vi "Actor Core.vi"(8 "error in":errorcluster, 11 "Power Meter Display in":refnum<class "Power Meter Display.lvclass">) -> (0 "error out":errorcluster, 3 "Actor out":refnum<class "Actor.lvclass">)   [LabVIEW 2013, in "Display Panel.lvlib" / "Power Meter Display.lvclass"]
doc: "(<B>Filename</B>: Actor Framework.lvlib:Actor.lvclass:Actor Core.vi)\n\nReceives messages to the actor, reacts to them, and initiates any error handling that may shut the actor down.\n\nDescendant classes may override this VI to append parallel tasks for the actor to complete while it handles messages. Overrides use the Call Parent Method node."
uses:
  Power Meter Display.lvclass
  <vilib>/ActorFramework/Actor/Actor.lvclass
  <vilib>/ActorFramework/Message Enqueuer/Message Priority.ctl
  Abstract Display/Abstract Display.lvclass/Abstract Display.ctl
  Power Meter Display.lvclass/Power Meter Display.ctl
  <vilib>/ActorFramework/Actor/Actor.lvclass/Actor.ctl
  Abstract Display/Abstract Display.lvclass
  <vilib>/ActorFramework/Message Enqueuer/Message Enqueuer.lvclass/Message Enqueuer.ctl
  Generic Instrument/Generic Card Messages/Write Data To Stop Bit Msg/Write Data To Stop Bit Msg.lvclass/Write Data To Stop Bit Msg.ctl
  <vilib>/ActorFramework/Message Enqueuer/Enqueue.vi
  <vilib>/ActorFramework/Message Enqueuer/Init from Existing Queue.vi
  <vilib>/ActorFramework/Message Priority Queue/Priority Enqueue.vi
  <vilib>/ActorFramework/Message Enqueuer/Message Enqueuer.lvclass
  Generic Instrument/Generic Card Messages/Write Data To Stop Bit Msg/Write Data To Stop Bit Msg.lvclass
  <vilib>/ActorFramework/Stop Msg/Stop Msg.lvclass
panel:
  out "Amp-Hour":dbl
  out "Start blinking":bool=TRUE
  out "Numeric Control":i32
  out "Blinker":bool caption="Warming"
  in  "EXit":bool
  in  "Stop":bool
  out "Time":dbl format="%<%H:%M:%S>t"
  out "Watt-Hour":dbl
  out "Frequency":dbl
  out "Power":dbl
  out "Current":dbl
  out "Voltage":dbl
  out "Card #":dbl
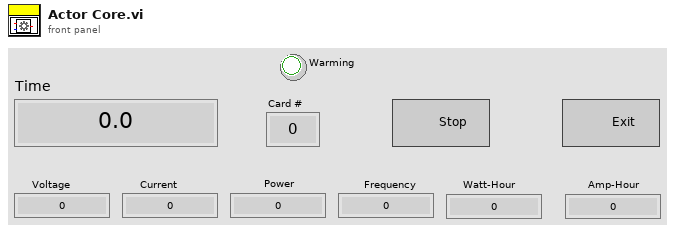
[diagram p1: front panel]
types:
  T1 = typedef "Actor Framework.lvlib/Message Enqueuer.lvclass/Message Priority.ctl" = enum16{"Low", "Normal", "High"}
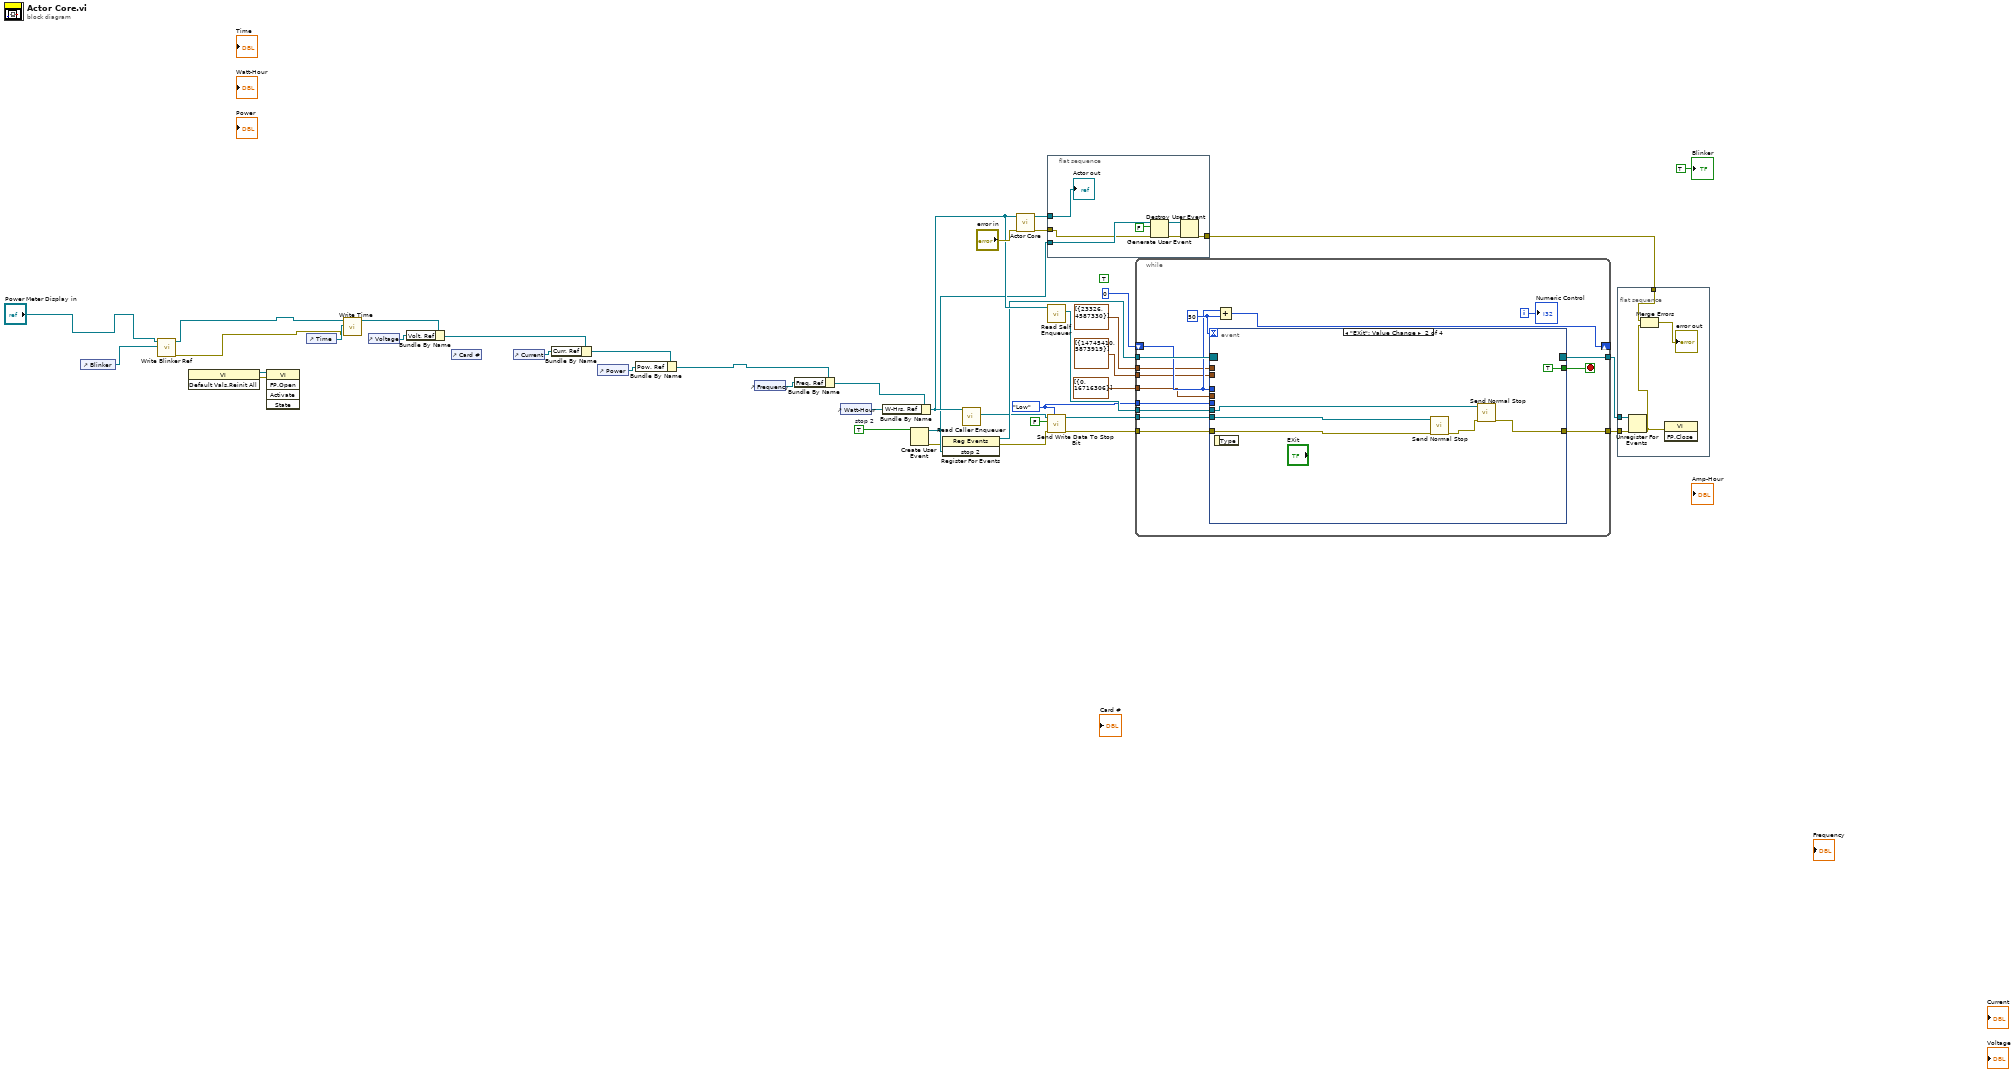
[diagram p0: block diagram]
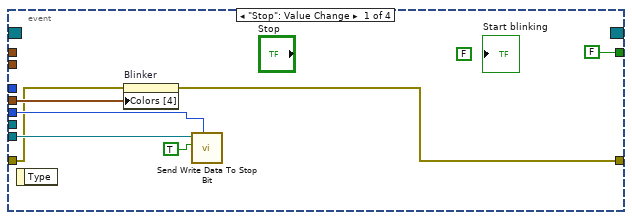
[diagram p2: hidden frame]
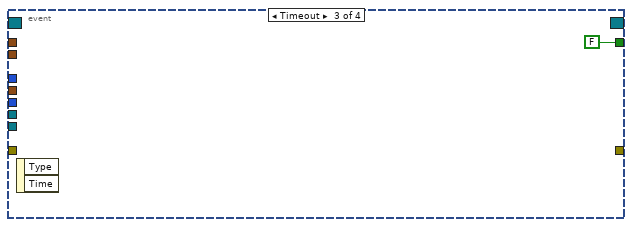
[diagram p3: hidden frame]
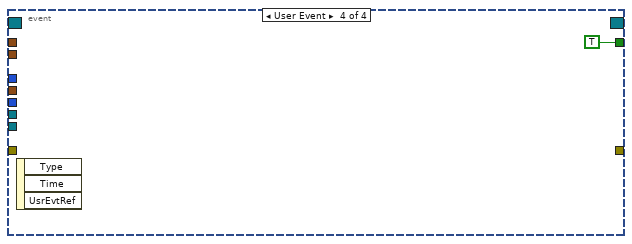
[diagram p4: hidden frame]
diagram:
  w13 = Message_Priority."Low" ("Message Priority (Normal)")
  (unwired) TRUE
  w21 = TRUE  # stop 2
  n1 = control-ref of="Blinker"() -> (w6:refnum<vi>)
  n2 = call "Write Blinker Ref.vi"("Blinker Ref"=w6, "Abstract Display in"="Power Meter Display in") -> ("error out"=w3:errorcluster, "Abstract Display out"=w4:refnum<class "Power Meter Display.lvclass">)  [unwired: 8 in]
  n3 = invoke class="VI" method="Default Vals.Reinit All"() -> (reference out=w27:refnum<vi>, error out=w12:errorcluster)  [unwired: 3 in, 1 out]
  n4 = invoke class="VI" method="FP.Open"(reference=w27, error in=w12) -> ()  [unwired: 3 in, 5 out]
  n5 = control-ref of="Time"() -> (w29:refnum<vi>)
  n6 = call "Write Time.vi"("error in (no error)"=w3, "Time"=w29, "Abstract Display in"=w4) -> ("Abstract Display out"=w30:refnum<class "Power Meter Display.lvclass">)  [unwired: 7 in, 1 out]
  n7 = control-ref of="Voltage"() -> (w38:refnum<vi>)
  n8 = Bundle By Name(cluster=w30, "Volt. Ref"=w38) -> (w1:refnum<class "Power Meter Display.lvclass">)
  n9 = control-ref of="Card #"() -> ()  [unwired: 1 out]
  n10 = control-ref of="Current"() -> (w34:refnum<vi>)
  n11 = Bundle By Name(cluster=w1, "Curr. Ref"=w34) -> (w36:refnum<class "Power Meter Display.lvclass">)
  n12 = control-ref of="Power"() -> (w33:refnum<vi>)
  n13 = Bundle By Name(cluster=w36, "Pow. Ref"=w33) -> (w5:refnum<class "Power Meter Display.lvclass">)
  n14 = control-ref of="Frequency"() -> (w32:refnum<vi>)
  n15 = Bundle By Name(cluster=w5, "Freq. Ref"=w32) -> (w35:refnum<class "Power Meter Display.lvclass">)
  n16 = control-ref of="Watt-Hour"() -> (w31:refnum<vi>)
  n17 = Bundle By Name(cluster=w35, "W-Hrs. Ref"=w31) -> (w26:refnum<class "Power Meter Display.lvclass">)
  n18 = Create User Event(user event datatype=w21) -> (user event=w22:refnum<user-event>, error out=w9:errorcluster)  [unwired: 1 in]
  n19 = register-events(error in=w9, w22) -> (reference out=w24:refnum<event-registration>, error out=w8:errorcluster)  [unwired: 1 in]
  n20 = call <vilib>:"Read Caller Enqueuer.vi"("Actor"=w26) -> ("Caller Enqueuer"=w16:refnum<class "Message Enqueuer.lvclass">)  [unwired: 10 in]
  n21 = call-parent "Actor Core.vi"("error in"="error in", "Abstract Display in"=w26) -> ("error out"=w40:errorcluster, "Actor out"=w39:refnum<class "Actor.lvclass">)  [unwired: 8 in]
  n22 = flat-sequence {
    tunnel: w40 -> [w43]
    tunnel: w39 -> [w47]
    tunnel: w22 -> [w46]
    tunnel: [w41] -> w7
    frame #0 {
      n23 = Generate User Event(user event=w46, event data cluster=FALSE ("event data"), error in=w43) -> (user event out=w44:refnum<user-event>, error out=w42:errorcluster)  [unwired: 1 in]
      n24 = Destroy User Event(user event=w44, error in=w42) -> (error out=w41:errorcluster)
      "Actor out" <- w47
    }
  }
  n25 = call <vilib>:"Read Self Enqueuer.vi"("Actor"=w26) -> ("Self Enqueuer"=w28:refnum<class "Message Enqueuer.lvclass">)  [unwired: 10 in]
  n26 = call "Send Write Data To Stop Bit.vi"("Message Priority (Normal)"=w13, "error in (no error)"=w8, "Stop Bit"=FALSE ("stop bit"), "Message Enqueuer"=w16) -> ("error out"=w10:errorcluster, "Message Enqueuer out"=w14:refnum<class "Message Enqueuer.lvclass">)  [unwired: 6 in]
  n27 = while {
    tunnel: w28 -> [w62]
    tunnel: w14 -> [w60]
    tunnel: cluster{u32, u32}[] [{0, 16716306}] ("Colors [4]") -> [w53]
    tunnel: w24 -> [w59]
    tunnel: [w58] -> w23
    shift-right: [w55] -> _
    shift-left: 0 -> [w54]
    tunnel: cluster{u32, u32}[] [{14745410, 5873919}] ("Colors [4]") -> [w52]
    tunnel: cluster{u32, u32}[] [{23326, 4587330}] ("Color 2 (Background, Foreground)") -> [w51]
    tunnel: w13 -> [w50]
    tunnel: [w49] -> w11
    tunnel: w10 -> [w48]
    i -> [w57]
    stop <- w61 stop-if-true
    w56 = 50
    n28 = event shown="[1] \"EXit\": Value Change" {
      selector: w59 -> [_ _ _ _]
      dyn-events: [_ _ _ _] -> w58
      timeout: w56 -> [_ _ _ _]
      tunnel: w62 -> [_ w70 _ _]
      tunnel: [FALSE TRUE FALSE TRUE] -> w61
      tunnel: w60 -> [w67 w74 _ _]
      tunnel: w53 -> [w69 _ _ _]
      tunnel: w54 -> [_ _ _ _]
      tunnel: w52 -> [_ _ _ _]
      tunnel: w51 -> [_ _ _ _]
      tunnel: w50 -> [w65 _ _ _]
      tunnel: [w63 w71 _ _] -> w49
      tunnel: w48 -> [w64 w73 _ _]
      event "Stop": Value Change {
        (unwired) FALSE ("stop blinking")
        n29 = event-data() -> ()  [unwired: 1 in, 1 out]
        n30 = property on="Blinker" class="Bool (strict)"(error in=w64, "Colors [4]"=w69) -> (error out=w63:errorcluster)  [unwired: 1 in, 1 out]
        n31 = call "Send Write Data To Stop Bit.vi"("Message Priority (Normal)"=w65, "Stop Bit"=TRUE ("stop bit"), "Message Enqueuer"=w67) -> ()  [unwired: 7 in, 2 out]
      }
      event "EXit": Value Change {
        n32 = event-data() -> ()  [unwired: 1 in, 1 out]
        n33 = call <vilib>:"Send Normal Stop.vi"("error in (no error)"=w73, "Message Enqueuer"=w74) -> ("error out"=w72:errorcluster)  [unwired: 9 in]
        n34 = call <vilib>:"Send Normal Stop.vi"("error in (no error)"=w72, "Message Enqueuer"=w70) -> ("error out"=w71:errorcluster)  [unwired: 9 in]
      }
      event Timeout {
        n35 = event-data() -> ()  [unwired: 1 in, 2 out]
      }
      event User Event {
        n36 = event-data() -> ()  [unwired: 1 in, 3 out]
      }
    }
    n37 = Add(x=w54, y=w56) -> (x+y=w55:i32)
    "Numeric Control" <- w57
  }
  n38 = flat-sequence {
    tunnel: w23 -> [w82]
    tunnel: w11 -> [w81]
    tunnel: w7 -> [w78]
    frame #0 {
      n39 = Unregister For Events(event registration refnum=w82, error in=w81) -> (error out=w80:errorcluster)
      n40 = Merge Errors(w78, w80) -> (→"error out":errorcluster)
      n41 = invoke class="VI" method="FP.Close"(error in=w80) -> ()  [unwired: 2 in, 3 out]
    }
  }
  "Blinker" <- TRUE ("Boolean")
